vi "Test Parse lvproj.vi"(11 "Test Case In":refnum<class "Parsing XML.lvclass">) -> (0 "error out":errorcluster, 3 "Test Case Out":refnum<class "Parsing XML.lvclass">)   [LabVIEW 2020, in "Parsing XML.lvclass"]
uses:
  Parsing XML.lvclass
  source/Classes/Item/Item.lvclass
  Parsing XML.lvclass/Parsing XML.ctl
  4993e8ee-a06a-463a-9684-69129f64d5ce.vi
  source/VI Properties Editor.lvlib
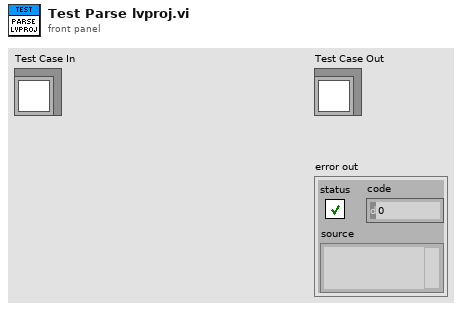
[diagram p1: front panel]
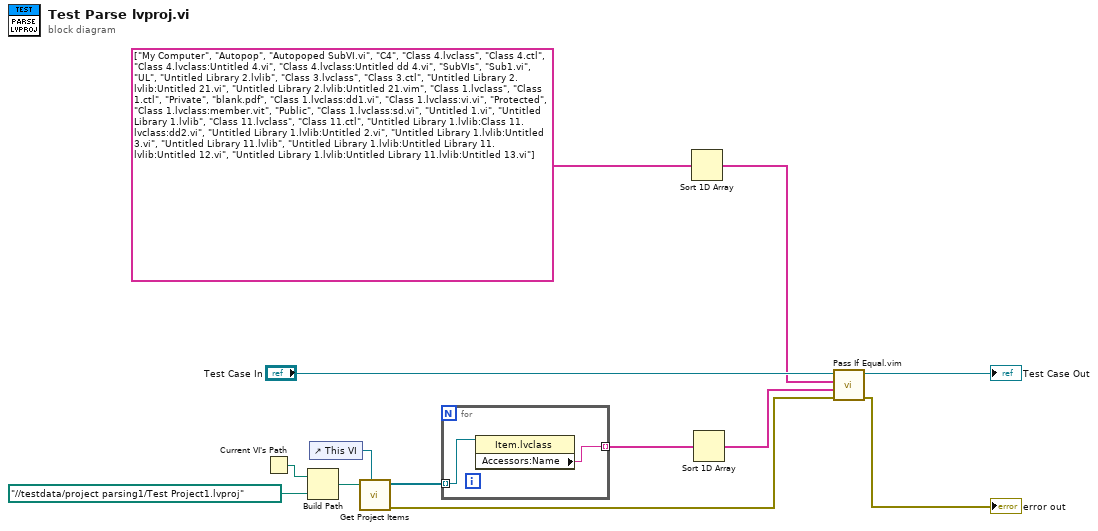
[diagram p0: block diagram]
diagram:
  n1 = Current VI's Path() -> (path=w10:path)
  n2 = Build Path(base path=w10, name or relative path=path "../../testdata/project parsing1/Test Project1.lvproj") -> (appended path=w5:path)
  n3 = control-ref of="This VI"() -> (w1:refnum<vi>)
  n4 = call "Get Project Items.vi"("Calling VI Ref"=w1, "Path"=w5) -> ("error out"=w9:errorcluster, "Items Data"=w8:refnum<class "Item.lvclass">[])  [unwired: 7 in, 1 out]
  n5 = for {
    tunnel: w8 -> [w15] mode=indexing
    tunnel: [w14] -> w7 mode=indexing
    n6 = property class="Item.lvclass"(reference=w15) -> ("Accessors:Name"=w14:string)  [unwired: 1 in, 2 out]
  }
  n7 = Sort 1D Array(array=string[] ["My Computer", "Autopop", "Autopoped SubVI.vi", "C4", "Class 4.lvclass", "Class 4.ctl", "Class 4.lvclass:Untitled 4.vi", "Class 4.lvclass:Untitled dd 4.vi", "SubVIs", "Sub1.vi", "UL", "Untitled Library 2.lvlib", "Class 3.lvclass", "Class 3.ctl", "Untitled Library 2.lvlib:Untitled 21.vi", "Untitled Library 2.lvlib:Untitled 21.vim", "Class 1.lvclass", "Class 1.ctl", "Private", "blank.pdf", "Class 1.lvclass:dd1.vi", "Class 1.lvclass:vi.vi", "Protected", "Class 1.lvclass:member.vit", "Public", "Class 1.lvclass:sd.vi", "Untitled 1.vi", "Untitled Library 1.lvlib", "Class 11.lvclass", "Class 11.ctl", "Untitled Library 1.lvlib:Class 11.lvclass:dd2.vi", "Untitled Library 1.lvlib:Untitled 2.vi", "Untitled Library 1.lvlib:Untitled 3.vi", "Untitled Library 11.lvlib", "Untitled Library 1.lvlib:Untitled Library 11.lvlib:Untitled 12.vi", "Untitled Library 1.lvlib:Untitled Library 11.lvlib:Untitled 13.vi"] ("Array")) -> (sorted array=w3:string[])
  n8 = Sort 1D Array(array=w7) -> (sorted array=w4:string[])
  n9 = call "Pass If Equal.vim"("error in (no error)"=w9, "Actual"=w4, "Expected"=w3, "LUnit Test Case In"="Test Case In") -> ("error out"=→"error out":errorcluster, "LUnit Test Case Out"=→"Test Case Out":refnum<class "Parsing XML.lvclass">)  [unwired: 6 in]
